vi "hdf5 read or write U16 array to dataset.vi"(4 "Chunk size":i32[](array[numeric])=[64, 64], 6 "Compression Level (0-disabled)":i32, 7 "File path":path=path "Test.hdf5", 8 "error in":errorcluster, 9 "Dataset name":string="test", 10 "Data to write":u16[][](array[numeric]), 11 "Operation":enum32{"Write", "Read"}(tab)) -> (0 "error out":errorcluster, 2 "write time":u32, 3 "Data read":u16[][](graph))   [LabVIEW 2018]
uses:
  <vilib>/UPVI/lvhdf5/dataset.llb/LVH5D Operation.ctl
  <vilib>/UPVI/lvhdf5/file.llb/LVH5F Operation.ctl
  <vilib>/Utility/miscctls.llb/LVRectTypeDef.ctl
  <vilib>/UPVI/lvhdf5/group.llb/H5G_obj_t.ctl
  <vilib>/UPVI/lvhdf5/utility.llb/Select HDF5 Dialog.vi
  <vilib>/UPVI/lvhdf5/utility.llb/Select HDF5 Dialog (Object Only).vi
  <vilib>/UPVI/lvhdf5/dataset.llb/Simple H5Dwrite (Variant).vi
  <vilib>/UPVI/lvhdf5/dataset.llb/Simple H5Dread (Variant).vi
  <vilib>/UPVI/lvhdf5/dataset.llb/Simple H5Dwrite.xnode
  <vilib>/UPVI/lvhdf5/library.llb/HDF5 Ref.ctl
  <vilib>/UPVI/lvhdf5/dataset.llb/Simple H5Dread.xnode
  <vilib>/UPVI/lvhdf5/identifier.llb/Not an HDF5 Refnum Constant.vi
  <vilib>/Utility/error.llb/Error Cluster From Error Code.vi
  <vilib>/UPVI/lvhdf5/dataspace.llb/H5Sselect_hyperslab.vi
  <vilib>/UPVI/lvhdf5/dataset.llb/H5Dget_space.vi
  <vilib>/UPVI/lvhdf5/dataspace.llb/H5Sclose.vi
  <vilib>/UPVI/lvhdf5/dataset.llb/H5Dclose.vi
  <vilib>/UPVI/lvhdf5/utility.llb/Select HDF5 Dialog (File and Object).vi
  <vilib>/UPVI/lvhdf5/dataset.llb/OpenCreateReplace Dataset by Element Type.vi
  <vilib>/UPVI/lvhdf5/dataset.llb/H5Dwrite (Variant).vi
  <vilib>/UPVI/lvhdf5/attribute.llb/private/LVH5AwriteWDTAttrs.vi
  <vilib>/UPVI/lvhdf5/dataset.llb/OpenCreateReplace Dataset.vi
  <vilib>/UPVI/lvhdf5/dataspace.llb/H5Sget_simple_extent_dims.vi
  <vilib>/UPVI/lvhdf5/dataset.llb/H5Dread (Variant).vi
  <vilib>/UPVI/lvhdf5/attribute.llb/private/LVH5AreadWDTAttrs.vi
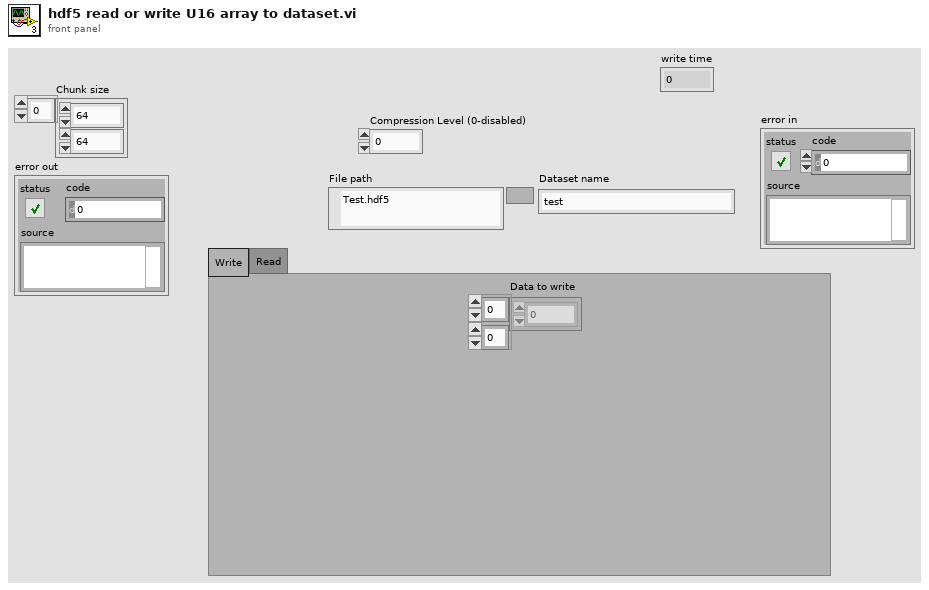
[diagram p1: front panel]
types:
  T1 = typedef "LVH5F Operation.ctl" = enum16{"open", "open or create", "create or replace", "create or replace (with confirmation)", "create", "open (read only)"}
  T2 = typedef "LVH5D Operation.ctl" = enum16{"open", "replace", "create", "open or create", "create or replace", "create or replace with confirmation"}
  T3 = typedef "LVRectTypeDef.ctl" = cluster{"Left":i16, "Top":i16, "Right":i16, "Bottom":i16}
  T4 = cluster{"Behavior":enum32{"Invalid", "Default", "Floating", "Floating/Auto-Hide", "Modal"}, "Position":T3, "Center":bool, "Title":string}
  T5 = typedef "H5G_obj_t.ctl" = i32
  T6 = cluster{"Object Types (any)":T5[], "Object Pattern":string}
  T7 = typedef "HDF5 Ref.ctl" = refnum<k1>
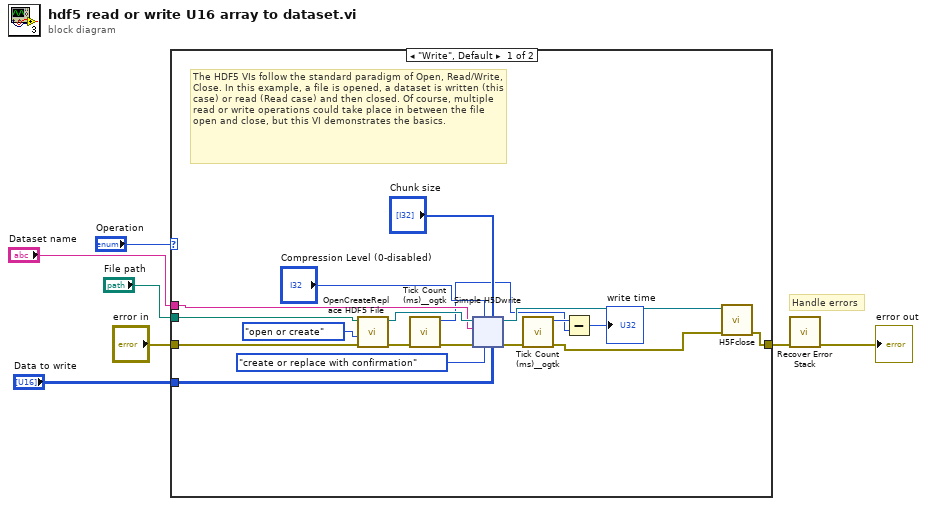
[diagram p0: block diagram]
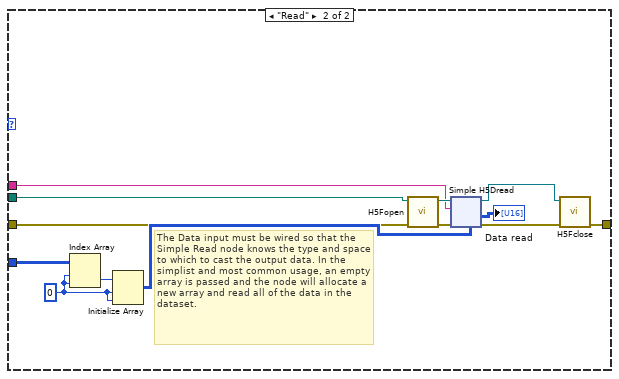
[diagram p2: hidden frame]
diagram:
  # "Handle errors"
  n1 = case shown="\"Write\", Default" "Operation" {
    tunnel: "File path" -> [w25 w240]
    tunnel: "Data to write" -> [w24 w236]
    tunnel: "Dataset name" -> [w17 w230]
    tunnel: "error in" -> [w23 w233]
    tunnel: [w18 w231] -> w5
    frame "Write", Default {
      # "The HDF5 VIs follow the standard paradigm of Open, Read/Write, Close. In this example, a file is opened, a dataset is written (this case) or read (Read case) and then closed. Of course, multiple read or write operations could take place in between the file open and close, but this VI demonstrates the basics."
      n2 = call <vilib>:"OpenCreateReplace HDF5 File.vi"("error in (no error)"=w23, "function (open or create)"=LVH5F_Operation."open or create", "path"=w25) -> ("error out"=w14:errorcluster, "HDF5 Ref out"=w22:T7)  [unwired: 5 in]
      n3 = call <userlib>:"Tick Count (ms)__ogtk.vi"("error in (no error)"=w14) -> ("error out"=w13:errorcluster, "millisecond timer value"=w10:u32)  [unwired: 9 in]
      n4 = xnode "Simple H5Dwrite"("Chunk size"="Chunk size", "Compression Level (0-disabled)"="Compression Level (0-disabled)", "Dataset Path"=w17, "error in (no error)"=w13, "operation (open or create)"=LVH5D_Operation."create or replace with confirmation", "HDF5 Path or Ref"=w22, "Data"=w24) -> ("HDF5 Ref out"=w19:T7, "error out"=w12:errorcluster)  [unwired: 1 in, 1 out]
      n5 = call <userlib>:"Tick Count (ms)__ogtk.vi"("error in (no error)"=w12) -> ("error out"=w8:errorcluster, "millisecond timer value"=w11:u32)  [unwired: 9 in]
      n6 = Subtract(x=w11, y=w10) -> (x-y=→"write time":u32)
      n7 = call <vilib>:"H5Fclose.vi"("error in (no error)"=w8, "HDF5 Ref"=w19) -> ("error out"=w18:errorcluster)  [unwired: 7 in]
    }
    frame "Read" {
      w228 = u16 0 ("index")
      # "The Data input must be wired so that the Simple Read node knows the type and space to which to cast the output data. In the simplist and most common usage, an empty array is passed and the node will allocate a new array and read all of the data in the dataset."
      n8 = Index Array(array=w236, index (row)=w228, index (col)=w228) -> (element=w235:u16)
      n9 = Initialize Array(w235, w228, w228) -> (w234:u16[][])
      n10 = call <vilib>:"H5Fopen.vi"("error in (no error)"=w233, "path"=w240) -> ("error out"=w239:errorcluster, "HDF5 Ref out"=w232:T7)  [unwired: 6 in]
      n11 = xnode "Simple H5Dread"("Dataset Path"=w230, "error in (no error)"=w239, "HDF5 Path or Ref"=w232, "Data"=w234) -> ("HDF5 Ref out"=w229:T7, "error out"=w237:errorcluster, "Data out"=→"Data read":u16[][])  [unwired: 1 out]
      n12 = call <vilib>:"H5Fclose.vi"("error in (no error)"=w237, "HDF5 Ref"=w229) -> ("error out"=w231:errorcluster)  [unwired: 7 in]
    }
  }
  n13 = call <vilib>:"Recover Error Stack.vi"("error in (no error)"=w5) -> ("error out"=→"error out":errorcluster)  [unwired: 5 in, 3 out]
